vi "RatchetReengage.vi"   [LabVIEW 2013]
uses:
  Robot Global Data.vi
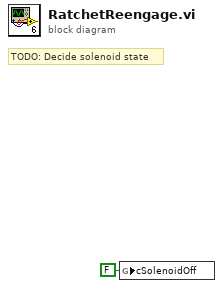
[diagram p0: block diagram]
diagram:
  # "TODO: Decide solenoid state"
  n1 = global write "Robot Global Data.vi" "cSolenoidOff"(FALSE ("cSolenoidOn")) -> ()
